vi "Update Registry BK shall be removed later.vi"() -> ()   [LabVIEW 2014]
uses:
  TypeDef/state.ctl
  TypeDef/Qmessage.ctl
  <vilib>/Utility/config.llb/Read Key (Path).vi
  <vilib>/Utility/file.llb/Read From Spreadsheet File (string).vi
  <vilib>/Utility/config.llb/Write Key (Path).vi
  <vilib>/Utility/config.llb/Read Key (String).vi
  <vilib>/Utility/config.llb/NI_LVConfig.lvlib
panel:
  out "ini file path":path
  in  "variation sheet":path caption="Variation Sheet (*.ini)"
  in  "Push":bool
  in  "Help Button":bool
  in  "Run":bool
  in  "Initialize":bool
  out "Status bar":string
  in  "Register change":bool
  in  "Add comment":bool
  in  "View":bool
  in  "NV 31":string
  in  "NV 30":string
  in  "NV 29":string
  in  "NV 28":string
  in  "NV 27":string
  in  "NV 26":string
  in  "NV 25":string
  in  "NV 24":string
  in  "NV 23":string
  in  "NV 22":string
  in  "NV 21":string
  in  "NV 20":string
  in  "NV 19":string
  in  "NV 18":string
  in  "NV 17":string
  in  "NV 16":string
  in  "NV 15":string
  in  "NV 14":string
  in  "NV 13":string
  in  "NV 12":string
  in  "NV 11":string
  in  "NV 10":string
  in  "NV 9":string
  in  "NV 8":string
  in  "NV 7":string
  in  "NV 6":string
  in  "NV 5":string
  in  "NV 4":string
  in  "NV 3":string
  in  "NV 2":string
  in  "NV 1":string
  out "V 31":string
  out "V 30":string
  out "V 29":string
  out "V 28":string
  out "V 27":string
  out "V 26":string
  out "V 25":string
  out "V 24":string
  out "V 23":string
  out "V 22":string
  out "V 21":string
  out "V 20":string
  out "V 19":string
  out "V 18":string
  out "V 17":string
  out "V 16":string
  out "V 15":string
  out "V 14":string
  out "V 13":string
  out "V 12":string
  out "V 11":string
  out "V 10":string
  out "V 9":string
  out "V 8":string
  out "V 7":string
  out "V 6":string
  out "V 5":string
  out "V 4":string
  out "V 3":string
  out "V 2":string
  out "V 1":string
  in  "tdms path":path caption="Variation Registry (*.tdms)"
  in  "Config Path":path caption="Config Path (*.txt)"
  out "N 31":string
  out "N 30":string
  out "N 29":string
  out "N 28":string
  out "N 27":string
  out "N 26":string
  out "N 25":string
  out "N 24":string
  out "N 23":string
  out "N 22":string
  out "N 21":string
  out "N 20":string
  out "N 19":string
  out "N 18":string
  out "N 17":string
  out "N 16":string
  out "N 15":string
  out "N 14":string
  out "N 13":string
  out "N 12":string
  out "N 11":string
  out "N 10":string
  out "N 9":string
  out "N 8":string
  out "N 7":string
  out "N 6":string
  out "N 5":string
  out "N 4":string
  out "N 3":string
  out "N 2":string
  out "N 1":string
  in  "Exit":bool
  # "Update Registry"
  # "Current Configuration"
  # "New Configuration"
  # "Component Name"
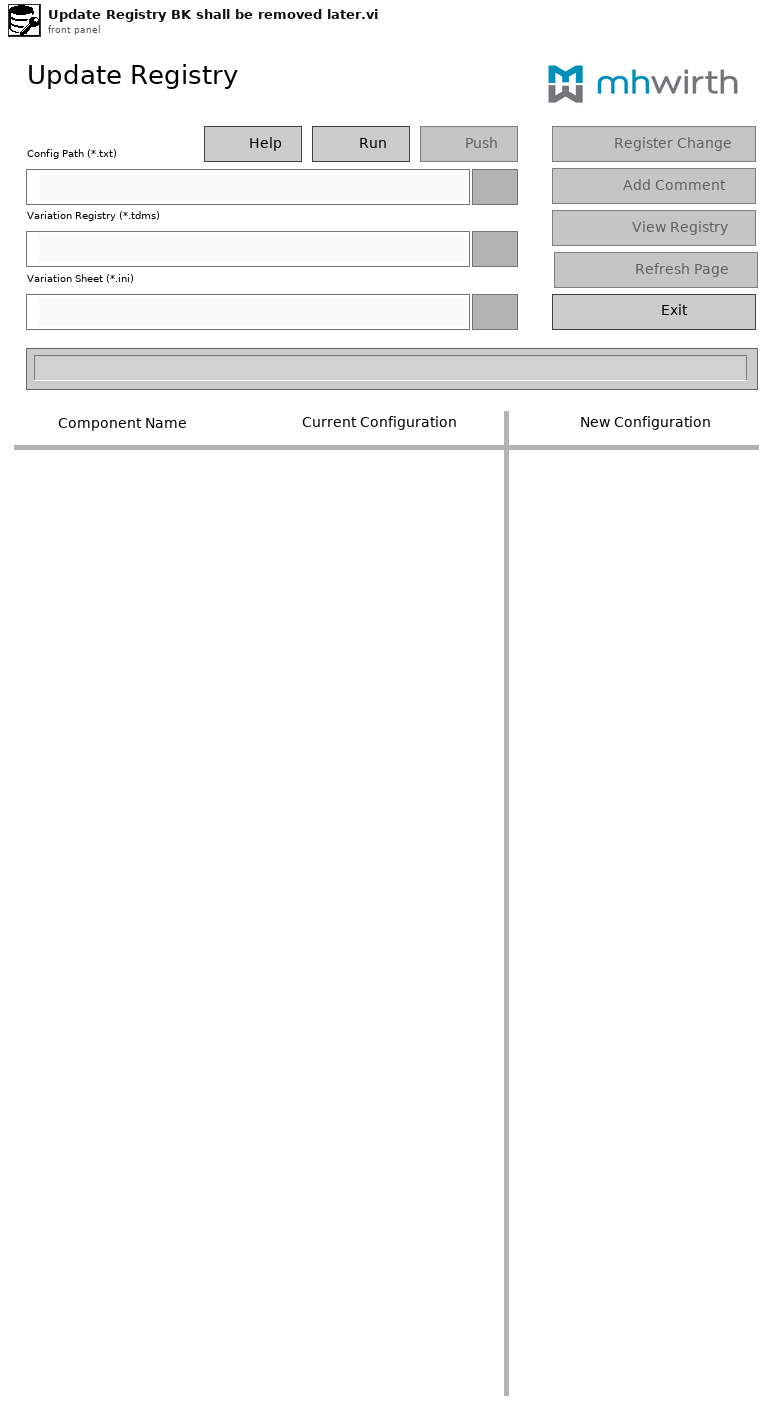
[diagram p1: front panel]
types:
  T1 = cluster{"Folder Path containing version information":path, "File name (including .ini)":path, "Section":string}
  T2 = typedef "Qmessage.ctl" = cluster{"data":variant, "state":T3}
  T3 = typedef "state.ctl" = enum16{"Run", "Initialize 1", "Initialize 2", "Read config file", "Read TDMS", "Config file Error", "Idle", "Update Comp Names", "Update Current Versions", "Make new configuration", "Register Change", "View Registry", "Add Comment", "No New Update", "Check current versions", "Read ini file", "Write ini file", "Read Variation Sheet", "Search and write current versions", "Close"}
  T4 = enum32{"invalid app kind", "Development System", "Run Time System", "Student Edition", "Embedded LabVIEW", "Evaluation", "Custom"}
  T5 = cluster{"keys":refnum<vi>[], "Names":refnum<vi>[], "Current Versions":refnum<vi>[], "New Versions":refnum<vi>[]}
  T6 = cluster{"path":path, "This VI":refnum<vi>, "Level of Application":u8}
  T7 = enum8{"Enabled", "Disabled", "Disabled and Grayed Out"}
  T8 = typedef "NI_LVConfig.lvlib/Config Data RefNum.ctl" = refnum<k1>
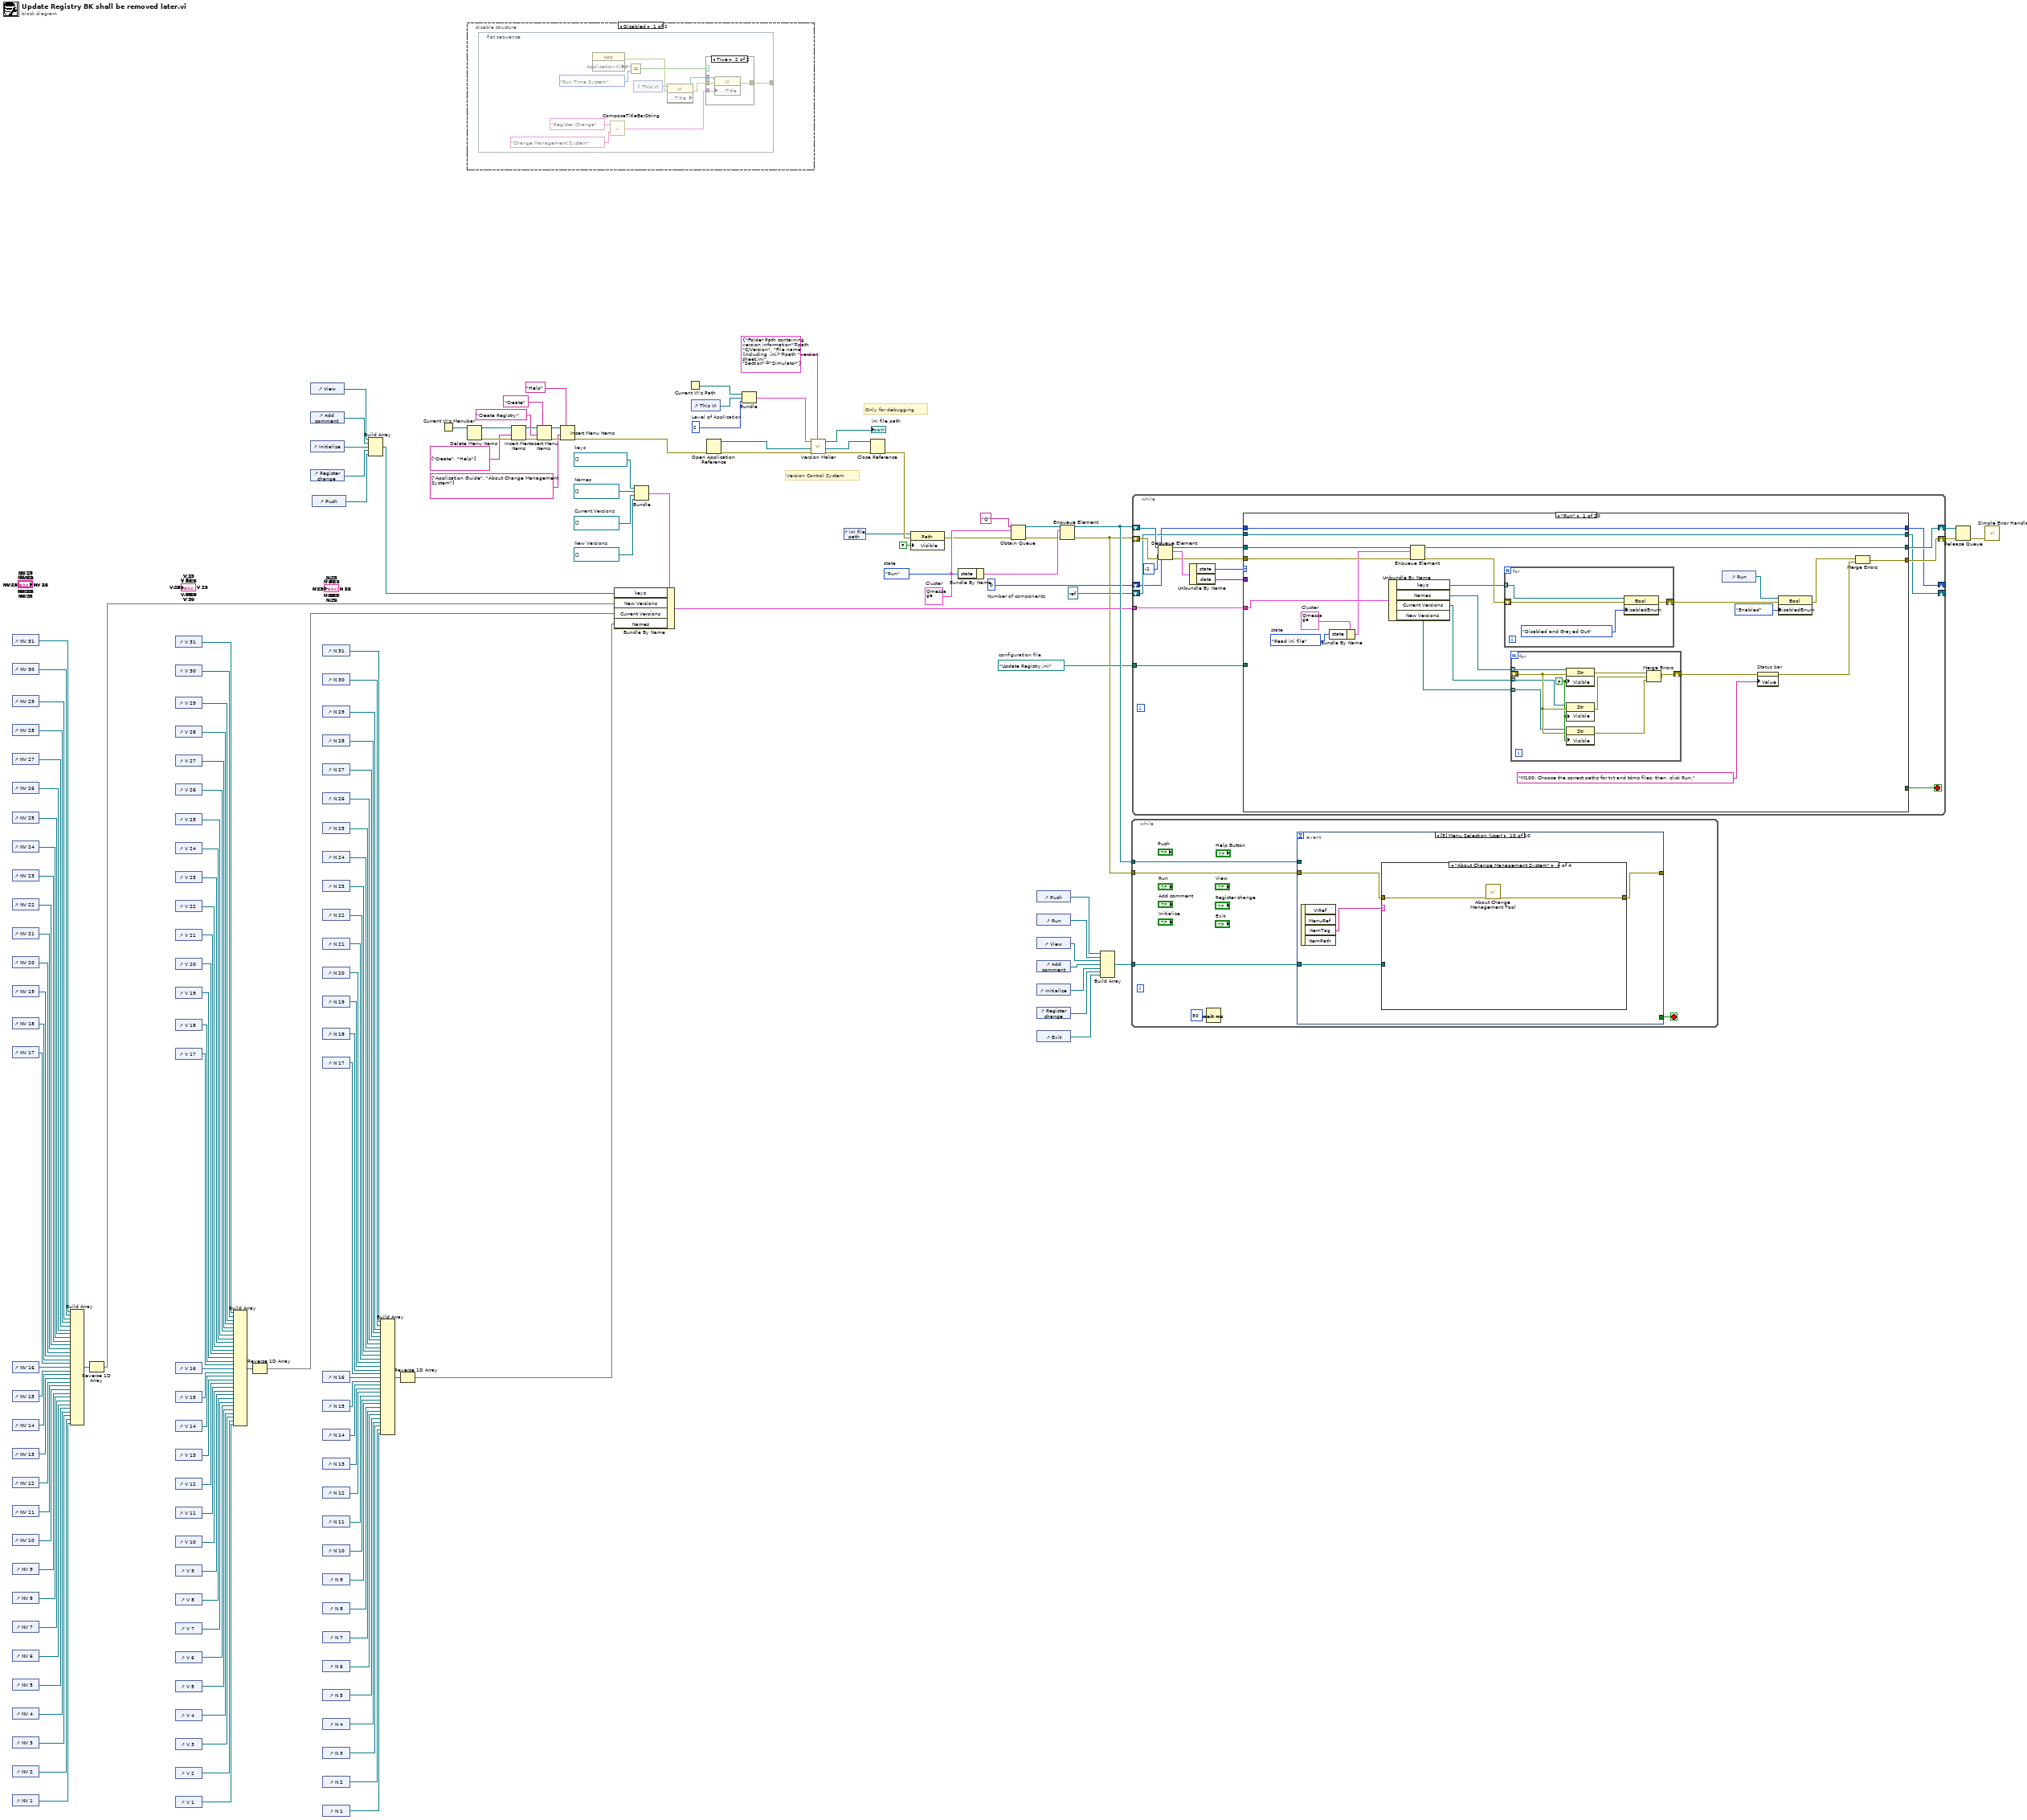
[diagram p0: block diagram]
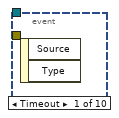
[diagram p4: hidden frame]
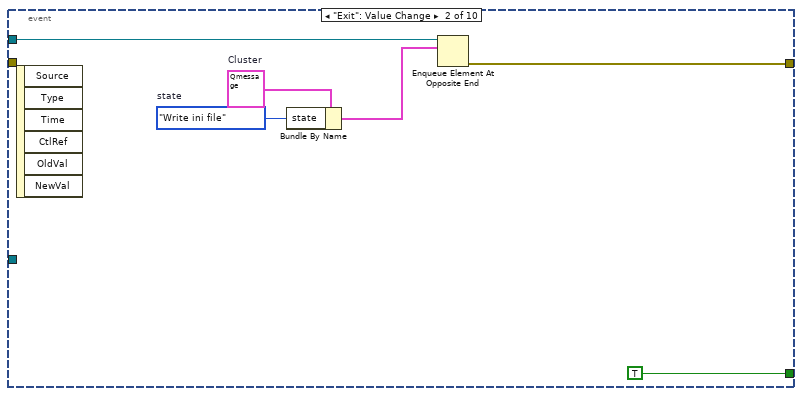
[diagram p5: hidden frame]
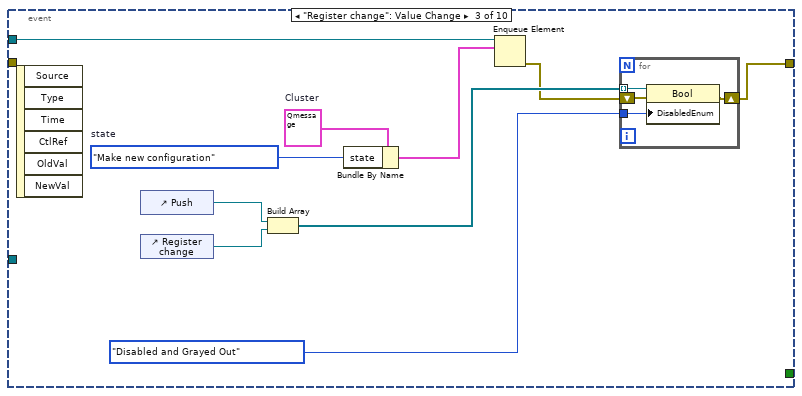
[diagram p6: hidden frame]
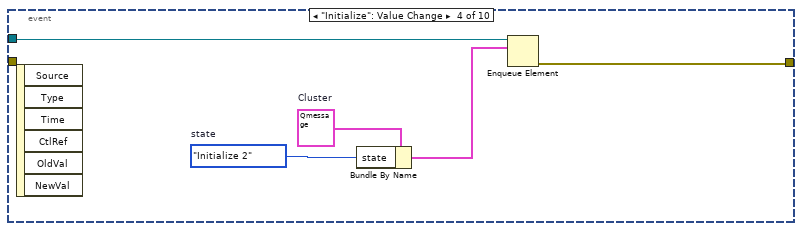
[diagram p7: hidden frame]
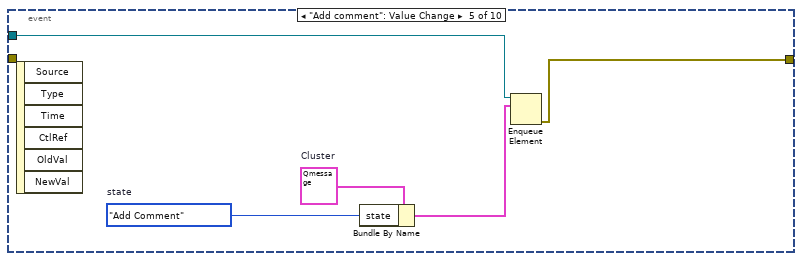
[diagram p8: hidden frame]
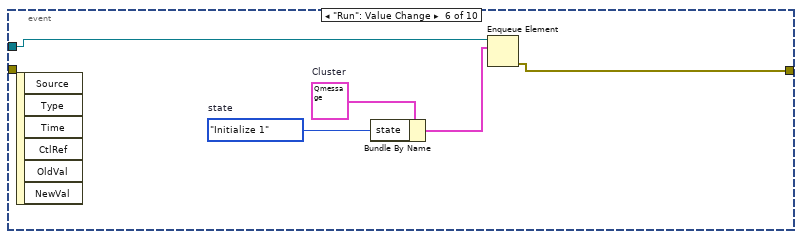
[diagram p9: hidden frame]
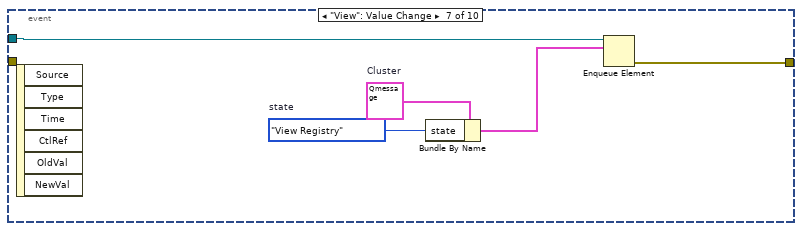
[diagram p10: hidden frame]
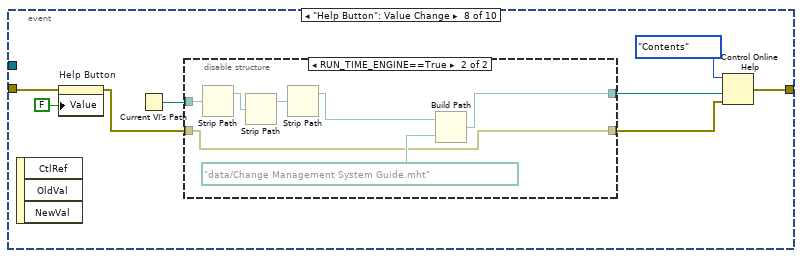
[diagram p11: hidden frame]
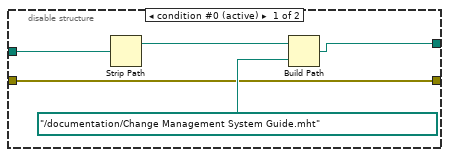
[diagram p12: hidden frame]
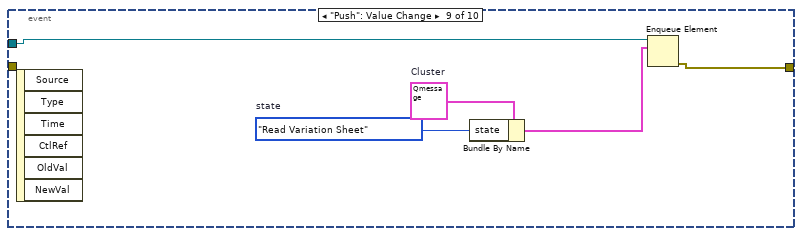
[diagram p13: hidden frame]
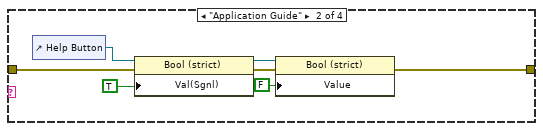
[diagram p15: hidden frame]
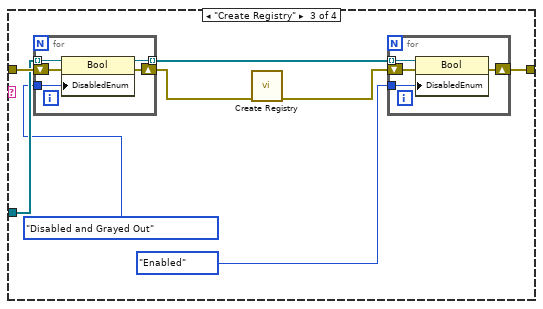
[diagram p16: hidden frame]
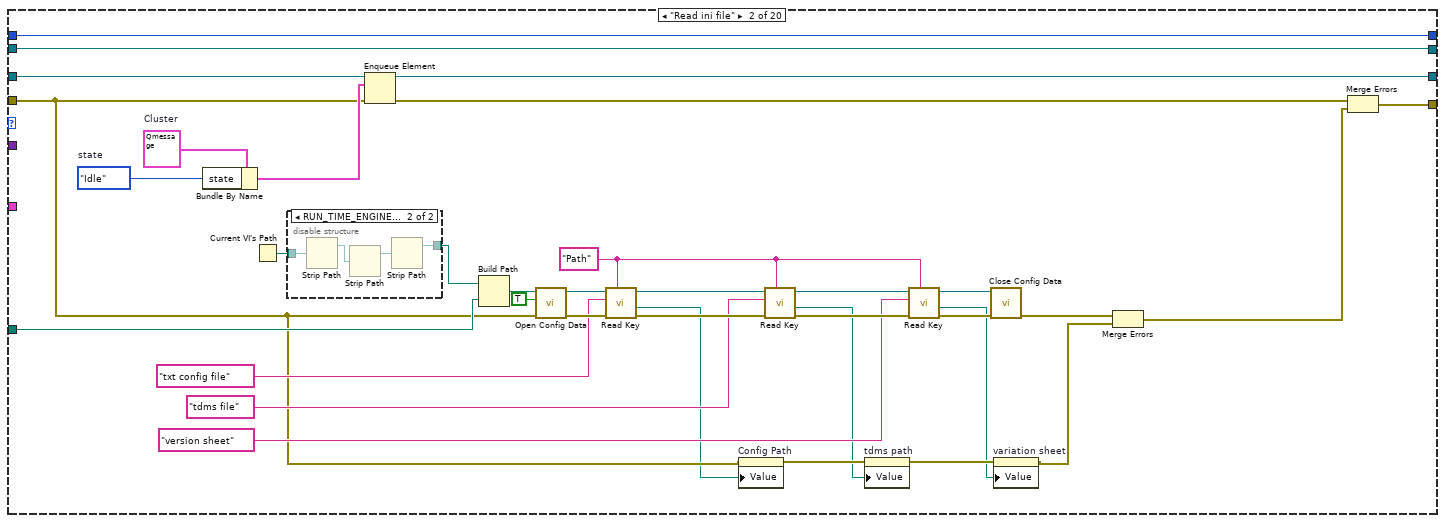
[diagram p17: hidden frame]
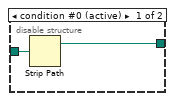
[diagram p18: hidden frame]
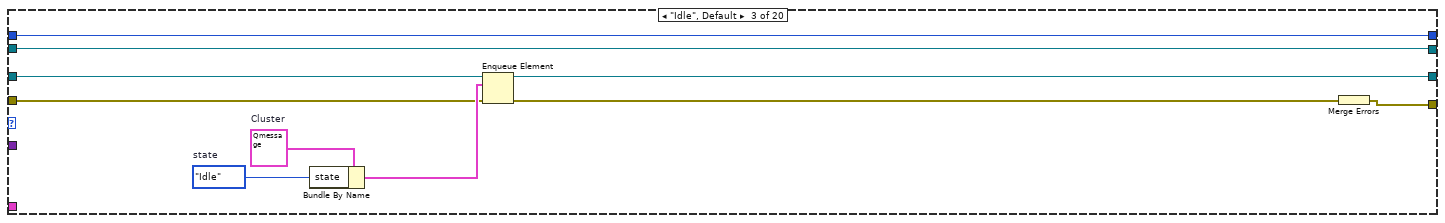
[diagram p19: hidden frame]
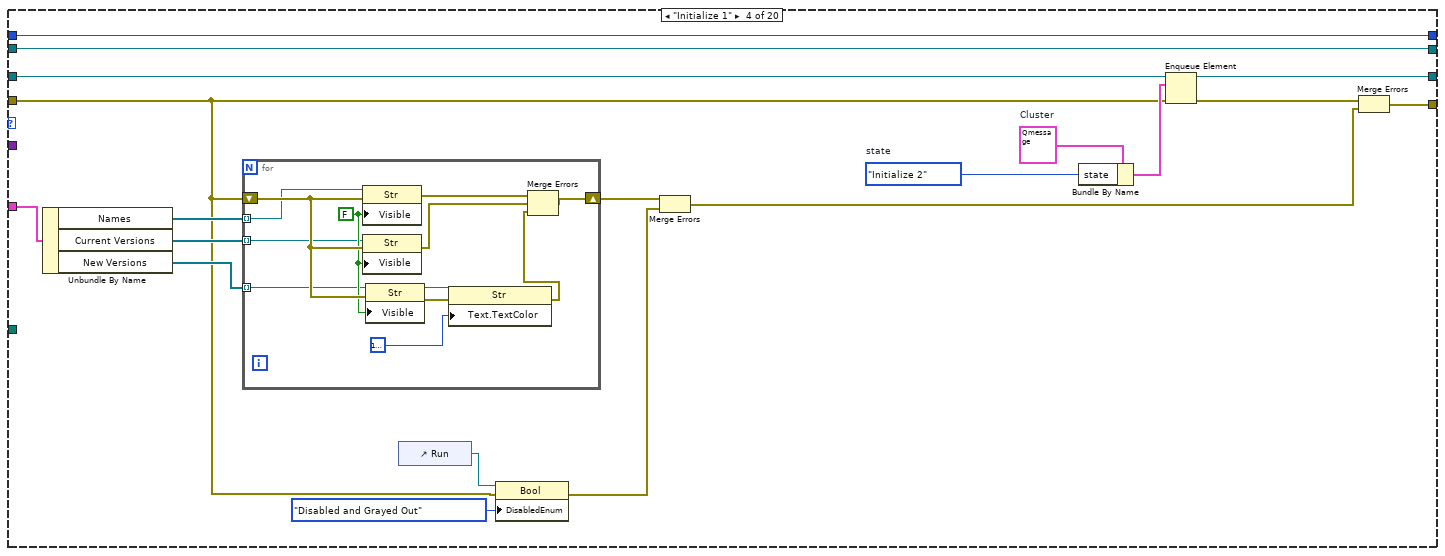
[diagram p20: hidden frame]
diagram:
  w25 = u8 2  # Level of Application
  w37 = path "Update Registry.ini"  # configuration file
  w52 = refnum<vi>[] []  # keys
  w57 = 0  # Number of components
  w49 = refnum<vi>[] []  # New Versions
  w50 = refnum<vi>[] []  # Current Versions
  w51 = refnum<vi>[] []  # Names
  w157 = T2 {"data"=variant, "state"=enum."Initialize 1"}  # Cluster
  w160 = state."Run"  # state
  # "Only for debugging"
  # "Version Control System"
  n1 = control-ref of="NV 31"() -> (w90:refnum<vi>)
  n2 = control-ref of="NV 30"() -> (w89:refnum<vi>)
  n3 = control-ref of="NV 29"() -> (w88:refnum<vi>)
  n4 = control-ref of="NV 28"() -> (w87:refnum<vi>)
  n5 = control-ref of="NV 27"() -> (w86:refnum<vi>)
  n6 = control-ref of="NV 26"() -> (w85:refnum<vi>)
  n7 = control-ref of="NV 25"() -> (w84:refnum<vi>)
  n8 = control-ref of="NV 24"() -> (w83:refnum<vi>)
  n9 = control-ref of="NV 23"() -> (w82:refnum<vi>)
  n10 = control-ref of="NV 22"() -> (w81:refnum<vi>)
  n11 = control-ref of="NV 21"() -> (w80:refnum<vi>)
  n12 = control-ref of="NV 20"() -> (w79:refnum<vi>)
  n13 = control-ref of="NV 19"() -> (w78:refnum<vi>)
  n14 = control-ref of="NV 18"() -> (w77:refnum<vi>)
  n15 = control-ref of="NV 17"() -> (w76:refnum<vi>)
  n16 = control-ref of="NV 16"() -> (w75:refnum<vi>)
  n17 = control-ref of="NV 15"() -> (w74:refnum<vi>)
  n18 = control-ref of="NV 14"() -> (w73:refnum<vi>)
  n19 = control-ref of="NV 13"() -> (w72:refnum<vi>)
  n20 = control-ref of="NV 12"() -> (w71:refnum<vi>)
  n21 = control-ref of="NV 11"() -> (w70:refnum<vi>)
  n22 = control-ref of="NV 10"() -> (w69:refnum<vi>)
  n23 = control-ref of="NV 9"() -> (w68:refnum<vi>)
  n24 = control-ref of="NV 8"() -> (w67:refnum<vi>)
  n25 = control-ref of="NV 7"() -> (w66:refnum<vi>)
  n26 = control-ref of="NV 6"() -> (w65:refnum<vi>)
  n27 = control-ref of="NV 5"() -> (w64:refnum<vi>)
  n28 = control-ref of="NV 4"() -> (w63:refnum<vi>)
  n29 = control-ref of="NV 3"() -> (w62:refnum<vi>)
  n30 = control-ref of="NV 2"() -> (w61:refnum<vi>)
  n31 = control-ref of="NV 1"() -> (w60:refnum<vi>)
  n32 = Build Array(w90, w89, w88, w87, w86, w85, w84, w83, w82, w81, w80, w79, w78, w77, w76, w75, w74, w73, w72, w71, w70, w69, w68, w67, w66, w65, w64, w63, w62, w61, w60) -> (w59:refnum<vi>[])
  n33 = Reverse 1D Array(array=w59) -> (reversed array=w43:refnum<vi>[])
  n34 = control-ref of="V 31"() -> (w122:refnum<vi>)
  n35 = control-ref of="V 30"() -> (w121:refnum<vi>)
  n36 = control-ref of="V 29"() -> (w120:refnum<vi>)
  n37 = control-ref of="V 28"() -> (w119:refnum<vi>)
  n38 = control-ref of="V 27"() -> (w118:refnum<vi>)
  n39 = control-ref of="V 26"() -> (w117:refnum<vi>)
  n40 = control-ref of="V 25"() -> (w116:refnum<vi>)
  n41 = control-ref of="V 24"() -> (w115:refnum<vi>)
  n42 = control-ref of="V 23"() -> (w114:refnum<vi>)
  n43 = control-ref of="V 22"() -> (w113:refnum<vi>)
  n44 = control-ref of="V 21"() -> (w112:refnum<vi>)
  n45 = control-ref of="V 20"() -> (w111:refnum<vi>)
  n46 = control-ref of="V 19"() -> (w110:refnum<vi>)
  n47 = control-ref of="V 18"() -> (w109:refnum<vi>)
  n48 = control-ref of="V 17"() -> (w108:refnum<vi>)
  n49 = control-ref of="V 16"() -> (w107:refnum<vi>)
  n50 = control-ref of="V 15"() -> (w106:refnum<vi>)
  n51 = control-ref of="V 14"() -> (w105:refnum<vi>)
  n52 = control-ref of="V 13"() -> (w104:refnum<vi>)
  n53 = control-ref of="V 12"() -> (w103:refnum<vi>)
  n54 = control-ref of="V 11"() -> (w102:refnum<vi>)
  n55 = control-ref of="V 10"() -> (w101:refnum<vi>)
  n56 = control-ref of="V 9"() -> (w100:refnum<vi>)
  n57 = control-ref of="V 8"() -> (w99:refnum<vi>)
  n58 = control-ref of="V 7"() -> (w98:refnum<vi>)
  n59 = control-ref of="V 6"() -> (w97:refnum<vi>)
  n60 = control-ref of="V 5"() -> (w96:refnum<vi>)
  n61 = control-ref of="V 4"() -> (w95:refnum<vi>)
  n62 = control-ref of="V 3"() -> (w94:refnum<vi>)
  n63 = control-ref of="V 2"() -> (w93:refnum<vi>)
  n64 = control-ref of="V 1"() -> (w92:refnum<vi>)
  n65 = Build Array(w122, w121, w120, w119, w118, w117, w116, w115, w114, w113, w112, w111, w110, w109, w108, w107, w106, w105, w104, w103, w102, w101, w100, w99, w98, w97, w96, w95, w94, w93, w92) -> (w91:refnum<vi>[])
  n66 = Reverse 1D Array(array=w91) -> (reversed array=w44:refnum<vi>[])
  n67 = control-ref of="View"() -> (w56:refnum<vi>)
  n68 = control-ref of="Add comment"() -> (w55:refnum<vi>)
  n69 = control-ref of="Initialize"() -> (w54:refnum<vi>)
  n70 = control-ref of="Register change"() -> (w53:refnum<vi>)
  n71 = control-ref of="Push"() -> (w38:refnum<vi>)
  n72 = control-ref of="N 31"() -> (w155:refnum<vi>)
  n73 = control-ref of="N 30"() -> (w154:refnum<vi>)
  n74 = control-ref of="N 29"() -> (w153:refnum<vi>)
  n75 = control-ref of="N 28"() -> (w152:refnum<vi>)
  n76 = control-ref of="N 27"() -> (w151:refnum<vi>)
  n77 = control-ref of="N 26"() -> (w150:refnum<vi>)
  n78 = control-ref of="N 25"() -> (w149:refnum<vi>)
  n79 = control-ref of="N 24"() -> (w148:refnum<vi>)
  n80 = control-ref of="N 23"() -> (w147:refnum<vi>)
  n81 = control-ref of="N 22"() -> (w146:refnum<vi>)
  n82 = control-ref of="N 21"() -> (w145:refnum<vi>)
  n83 = control-ref of="N 20"() -> (w144:refnum<vi>)
  n84 = control-ref of="N 19"() -> (w143:refnum<vi>)
  n85 = control-ref of="N 18"() -> (w142:refnum<vi>)
  n86 = control-ref of="N 17"() -> (w141:refnum<vi>)
  n87 = control-ref of="N 16"() -> (w140:refnum<vi>)
  n88 = control-ref of="N 15"() -> (w139:refnum<vi>)
  n89 = control-ref of="N 14"() -> (w138:refnum<vi>)
  n90 = control-ref of="N 13"() -> (w137:refnum<vi>)
  n91 = control-ref of="N 12"() -> (w136:refnum<vi>)
  n92 = control-ref of="N 11"() -> (w135:refnum<vi>)
  n93 = control-ref of="N 10"() -> (w134:refnum<vi>)
  n94 = control-ref of="N 9"() -> (w133:refnum<vi>)
  n95 = control-ref of="N 8"() -> (w132:refnum<vi>)
  n96 = control-ref of="N 7"() -> (w131:refnum<vi>)
  n97 = control-ref of="N 6"() -> (w130:refnum<vi>)
  n98 = control-ref of="N 5"() -> (w129:refnum<vi>)
  n99 = control-ref of="N 4"() -> (w128:refnum<vi>)
  n100 = control-ref of="N 3"() -> (w127:refnum<vi>)
  n101 = control-ref of="N 2"() -> (w126:refnum<vi>)
  n102 = control-ref of="N 1"() -> (w125:refnum<vi>)
  n103 = Build Array(w56, w55, w54, w53, w38) -> (w46:refnum<vi>[])
  n104 = Build Array(w155, w154, w153, w152, w151, w150, w149, w148, w147, w146, w145, w144, w143, w142, w141, w140, w139, w138, w137, w136, w135, w134, w133, w132, w131, w130, w129, w128, w127, w126, w125) -> (w124:refnum<vi>[])
  n105 = Reverse 1D Array(array=w124) -> (reversed array=w45:refnum<vi>[])
  n106 = Current VI's Menubar() -> (w22:refnum<k9>)
  n107 = disable-structure shown="Disabled" {
    frame Disabled {
      n108 = flat-sequence {
        tunnel: [w161] -> _
        frame #0 {
          n109 = property on="Property Node" class="App"() -> (error out=w163:errorcluster, "Application:Kind"=w169:T4)  [unwired: 2 in, 1 out]
          n110 = call "ComposeTitleBarString.vi"("ProjectName"="Change Management System" ("Application"), "Application"="Register Change") -> ("TitleBar"=w171:string)
          n111 = Equal?(x=w169, y=T4."Run Time System" ("Applikation:Typ")) -> (x = y?=w170:bool)
          n112 = control-ref of="This VI"() -> (w167:refnum<vi>)
          n113 = property on="Property Node" class="VI" props=["Front Panel.Title"](reference=w167, error in=w163) -> (reference out=w166:refnum<vi>, error out=w162:errorcluster)  [unwired: 1 out]
          n114 = case shown="True" w170 {
            tunnel: w171 -> [_ w176]
            tunnel: w166 -> [_ w175]
            tunnel: w162 -> [w172 w174]
            tunnel: [w172 w173] -> w161
            frame False {
            }
            frame True {
              n115 = property class="VI"(reference=w175, error in=w174, "Front Panel.Title"=w176) -> (error out=w173:errorcluster)  [unwired: 1 out]
            }
          }
        }
      }
    }
    frame Enabled {
    }
  }
  n116 = Delete Menu Items(9:w22) -> (0:w21:errorcluster, 3:w20:refnum<k9>)  [unwired: 3 in]
  n117 = Insert Menu Items(6:w21, 7:string[] ["Create", "Help"] ("item tags"), 9:w20) -> (0:w16:errorcluster, 3:w18:refnum<k9>)  [unwired: 3 in, 1 out]
  n118 = Insert Menu Items(5:"Create", 6:w16, 7:"Create Registry", 9:w18) -> (0:w15:errorcluster, 3:w14:refnum<k9>)  [unwired: 2 in, 1 out]
  n119 = Insert Menu Items(5:"Help", 6:w15, 7:string[] ["Application Guide", "About Change Management System"] ("item tags"), 9:w14) -> (0:w10:errorcluster)  [unwired: 2 in, 2 out]
  n120 = Bundle("keys"=w52, "Names"=w51, "Current Versions"=w50, "New Versions"=w49) -> (w47:T5)  [unwired: 1 in]
  n121 = Bundle By Name(cluster=w47, "keys"=w46, "New Versions"=w43, "Current Versions"=w44, "Names"=w45) -> (w48:T5)
  n122 = Current VI's Path() -> (path=w23:path)
  n123 = control-ref of="This VI"() -> (w24:refnum<vi>)
  n124 = Open Application Reference(8:w10) -> (0:w36:errorcluster, 3:w32:refnum<vi>)  [unwired: 3 in]
  n125 = Bundle("path"=w23, "This VI"=w24, "Level of Application"=w25) -> (w26:T6)  [unwired: 1 in]
  n126 = call "Version Maker.vi"("Version Sheet Cluster"=T1 {"Folder Path containing version information"=path "C:/Version", "File name (including .ini)"=path "version sheet.ini", "Section"="Simulator"}, "Error In"=w36, "Open Application Reference in"=w32, "VI Information"=w26) -> ("Error Out"=w35:errorcluster, "Open Application Reference out"=w31:refnum<vi>, "ini file path"=→"ini file path":path)  [unwired: 5 in]
  n127 = control-ref of="ini file path"() -> (w28:refnum<vi>)
  n128 = Close Reference(reference=w31, error in (no error)=w35) -> (error out=w29:errorcluster)
  n129 = property class="Path"(reference=w28, error in=w29, "Visible"=FALSE) -> (error out=w30:errorcluster)  [unwired: 1 out]
  n130 = Bundle By Name(cluster=w157, "state"=w160) -> (w156:T2)
  n131 = Obtain Queue(name (unnamed)="Q", element data type=w157, error in (no error)=w30) -> (queue out=w159:refnum<queue>, error out=w42:errorcluster)  [unwired: 2 in, 1 out]
  n132 = control-ref of="Push"() -> (w8:refnum<vi>)
  n133 = control-ref of="Run"() -> (w7:refnum<vi>)
  n134 = control-ref of="View"() -> (w6:refnum<vi>)
  n135 = control-ref of="Add comment"() -> (w5:refnum<vi>)
  n136 = control-ref of="Initialize"() -> (w4:refnum<vi>)
  n137 = control-ref of="Register change"() -> (w3:refnum<vi>)
  n138 = control-ref of="Exit"() -> (w2:refnum<vi>)
  n139 = Enqueue Element(queue=w159, element=w156, error in (no error)=w42) -> (queue out=w123:refnum<queue>, error out=w9:errorcluster)  [unwired: 1 in, 1 out]
  n140 = Build Array(w8, w7, w6, w5, w4, w3, w2) -> (w1:refnum<vi>[])
  n141 = while {
    tunnel: w123 -> [w180]
    tunnel: w9 -> [w178]
    tunnel: w1 -> [w177]
    stop <- w179 stop-if-true
    n142 = Wait (ms)(milliseconds to wait=u32 50) -> ()  [unwired: 1 out]
    n143 = event shown="[9] Menu Selection (User)" {
      selector: _ -> [_ _ _ _ _ _ _ _ _ _]
      dyn-events: _ -> [_ _ _ _ _ _ _ _ _ _]
      timeout: _ -> [_ _ _ _ _ _ _ _ _ _]
      tunnel: w180 -> [_ w184 w195 w203 w211 w214 w218 _ w243 _]
      tunnel: [_ TRUE _ _ _ _ _ _ _ _] -> w179
      tunnel: [_ w182 w188 w202 w207 w212 w217 w228 w242 w248] -> _
      tunnel: w178 -> [_ _ _ _ _ _ _ w224 _ w249]
      tunnel: w177 -> [_ _ _ _ _ _ _ _ _ w247]
      event Timeout {
        n144 = event-data() -> ()  [unwired: 1 in, 2 out]
      }
      event "Exit": Value Change {
        w187 = T2 {"data"=variant, "state"=enum."Initialize 1"}  # Cluster
        w186 = state."Write ini file"  # state
        n145 = event-data() -> ()  [unwired: 1 in, 6 out]
        n146 = Bundle By Name(cluster=w187, "state"=w186) -> (w185:T2)
        n147 = Enqueue Element At Opposite End(queue=w184, element=w185) -> (error out=w182:errorcluster)  [unwired: 2 in, 2 out]
      }
      event "Register change": Value Change {
        w197 = T2 {"data"=variant, "state"=enum."Initialize 1"}  # Cluster
        w194 = state."Make new configuration"  # state
        n148 = event-data() -> ()  [unwired: 1 in, 6 out]
        n149 = control-ref of="Push"() -> (w193:refnum<vi>)
        n150 = control-ref of="Register change"() -> (w192:refnum<vi>)
        n151 = Build Array(w193, w192) -> (w191:refnum<vi>[])
        n152 = Bundle By Name(cluster=w197, "state"=w194) -> (w196:T2)
        n153 = Enqueue Element(queue=w195, element=w196) -> (error out=w189:errorcluster)  [unwired: 2 in, 2 out]
        n154 = for {
          tunnel: w191 -> [w201] mode=indexing
          tunnel: T7."Disabled and Grayed Out" ("Disabled") -> [w200]
          shift-right: [w198] -> w188
          shift-left: w189 -> [w199]
          n155 = property class="Bool"(reference=w201, error in=w199, "DisabledEnum"=w200) -> (error out=w198:errorcluster)  [unwired: 1 out]
        }
      }
      event "Initialize": Value Change {
        w206 = T2 {"data"=variant, "state"=enum."Initialize 1"}  # Cluster
        w204 = state."Initialize 2"  # state
        n156 = event-data() -> ()  [unwired: 1 in, 6 out]
        n157 = Bundle By Name(cluster=w206, "state"=w204) -> (w205:T2)
        n158 = Enqueue Element(queue=w203, element=w205) -> (error out=w202:errorcluster)  [unwired: 2 in, 2 out]
      }
      event "Add comment": Value Change {
        w209 = T2 {"data"=variant, "state"=enum."Initialize 1"}  # Cluster
        w208 = state."Add Comment"  # state
        n159 = event-data() -> ()  [unwired: 1 in, 6 out]
        n160 = Bundle By Name(cluster=w209, "state"=w208) -> (w210:T2)
        n161 = Enqueue Element(queue=w211, element=w210) -> (error out=w207:errorcluster)  [unwired: 2 in, 2 out]
      }
      event "Run": Value Change {
        w216 = T2 {"data"=variant, "state"=enum."Initialize 1"}  # Cluster
        w215 = state."Initialize 1"  # state
        n162 = event-data() -> ()  [unwired: 1 in, 6 out]
        n163 = Bundle By Name(cluster=w216, "state"=w215) -> (w213:T2)
        n164 = Enqueue Element(queue=w214, element=w213) -> (error out=w212:errorcluster)  [unwired: 2 in, 2 out]
      }
      event "View": Value Change {
        w221 = T2 {"data"=variant, "state"=enum."Initialize 1"}  # Cluster
        w220 = state."View Registry"  # state
        n165 = event-data() -> ()  [unwired: 1 in, 6 out]
        n166 = Bundle By Name(cluster=w221, "state"=w220) -> (w219:T2)
        n167 = Enqueue Element(queue=w218, element=w219) -> (error out=w217:errorcluster)  [unwired: 2 in, 2 out]
      }
      event "Help Button": Value Change {
        n168 = event-data() -> ()  [unwired: 1 in, 3 out]
        n169 = property on="Help Button" class="Bool (strict)"(error in=w224, "Value"=FALSE ("Help Button")) -> (error out=w223:errorcluster)  [unwired: 1 in, 1 out]
        n170 = Current VI's Path() -> (path=w227:path)
        n171 = disable-structure shown="RUN_TIME_ENGINE==True" {
          disable-tunnel: w227 -> [w234 w241]
          disable-tunnel: [w231 w237] -> w226
          disable-tunnel: w223 -> [w230 w235]
          disable-tunnel: [w230 w235] -> w222
          frame condition #0 (active) {
            n172 = Strip Path(path=w234) -> (stripped path=w233:path)  [unwired: 1 out]
            n173 = Build Path(base path=w233, name or relative path=path "../documentation/Change Management System Guide.mht") -> (appended path=w231:path)
          }
          frame condition #1 {
            n174 = Strip Path(path=w241) -> (stripped path=w240:path)  [unwired: 1 out]
            n175 = Strip Path(path=w240) -> (stripped path=w239:path)  [unwired: 1 out]
            n176 = Strip Path(path=w239) -> (stripped path=w236:path)  [unwired: 1 out]
            n177 = Build Path(base path=w236, name or relative path=path "data/Change Management System Guide.mht") -> (appended path=w237:path)
          }
        }
        n178 = Control Online Help(1:w222, 2:w226, 4:enum16{"Contents", "Key", "Close"}."Contents" ("Operation")) -> (0:w228:errorcluster)  [unwired: 1 in]
      }
      event "Push": Value Change {
        w246 = T2 {"data"=variant, "state"=enum."Initialize 1"}  # Cluster
        w245 = state."Read Variation Sheet"  # state
        n179 = event-data() -> ()  [unwired: 1 in, 6 out]
        n180 = Bundle By Name(cluster=w246, "state"=w245) -> (w244:T2)
        n181 = Enqueue Element(queue=w243, element=w244) -> (error out=w242:errorcluster)  [unwired: 2 in, 2 out]
      }
      event Menu Selection (User) {
        n182 = event-data() -> ("ItemTag"=w250:string)  [unwired: 1 in, 3 out]
        n183 = case shown="\"About Change Management System\"" w250 {
          tunnel: w249 -> [w251 w253 w266 w277]
          tunnel: [w251 w252 w259 w276] -> w248
          tunnel: w247 -> [_ _ w265 _]
          frame "default", Default {
          }
          frame "Application Guide" {
            n184 = control-ref of="Help Button"() -> (w258:refnum<vi>)
            n185 = property class="Bool (strict)"(reference=w258, error in=w253, "Val(Sgnl)"=TRUE) -> (reference out=w256:refnum<vi>, error out=w255:errorcluster)
            n186 = property class="Bool (strict)"(reference=w256, error in=w255, "Value"=FALSE ("Value (Signaling)")) -> (error out=w252:errorcluster)  [unwired: 1 out]
          }
          frame "Create Registry" {
            n187 = for {
              tunnel: w265 -> [w274] mode=indexing
              tunnel: T7."Disabled and Grayed Out" ("Disabled") -> [w273]
              tunnel: [w272] -> w263 mode=indexing
              shift-right: [w271] -> w261
              shift-left: w266 -> [w275]
              n188 = property class="Bool"(reference=w274, error in=w275, "DisabledEnum"=w273) -> (reference out=w272:refnum<vi>, error out=w271:errorcluster)
            }
            n189 = call "Create Registry.vi"("Error In"=w261) -> ("Error Out"=w260:errorcluster)  [unwired: 10 in]
            n190 = for {
              tunnel: w263 -> [w269] mode=indexing
              tunnel: T7."Enabled" ("Disabled") -> [w268]
              shift-right: [w267] -> w259
              shift-left: w260 -> [w270]
              n191 = property class="Bool"(reference=w269, error in=w270, "DisabledEnum"=w268) -> (error out=w267:errorcluster)  [unwired: 1 out]
            }
          }
          frame "About Change Management System" {
            n192 = call "About Change Management Tool.vi"("Error In"=w277) -> ("Error Out"=w276:errorcluster)  [unwired: 10 in]
          }
        }
      }
    }
  }
  n193 = while {
    shift-right: [w288] -> w40
    shift-left: w123 -> [w292]
    shift-right: [w287] -> w41
    shift-left: w9 -> [w294]
    tunnel: w48 -> [w283]
    shift-right: [w282] -> _
    shift-left: refnum<k34> refnum ("tdms file out") -> [w281]
    shift-right: [w280] -> _
    shift-left: w57 -> [w279]
    tunnel: w37 -> [w278]
    stop <- w284 stop-if-true
    n194 = Dequeue Element(queue=w292, timeout in ms (-1)=-1, error in (no error)=w294) -> (queue out=w289:refnum<queue>, element=w293:T2, error out=w285:errorcluster)  [unwired: 1 out]
    n195 = Unbundle By Name(w293) -> ("state"=w291:T3, "data"=w290:variant)
    n196 = case shown="\"Run\"" w291 {
      tunnel: w290 -> [_ _ _ _ _ _ _ w526 w549 _ w633 _ _ _ _ _ _ _ _ w862]
      tunnel: w289 -> [w299 w362 w376 w382 w421 w439 w475 w518 w542 w576 w627 w662 w688 w704 w720 w732 w760 w803 w822 w864]
      tunnel: [w298 w361 w375 w381 w420 w438 w475 w518 w542 w576 w627 w662 w688 w704 w720 w732 w759 w803 w821 w864] -> w288
      tunnel: w285 -> [w297 w336 w373 w385 w415 w441 w474 w523 w546 w585 w632 w667 w682 w707 w715 w738 w758 w794 w820 w853]
      tunnel: [w309 w356 w372 w394 w427 w449 w477 w517 w541 w578 w628 w659 w679 w703 w714 w738 w763 w800 w819 w852] -> w287
      tunnel: [_ _ _ _ _ _ _ _ _ _ _ _ _ _ _ _ _ TRUE _ _] -> w284
      tunnel: w283 -> [w314 _ _ w399 w416 _ _ w513 w540 w588 _ _ _ _ w717 _ _ w789 _ w858]
      tunnel: [w316 w364 w380 w389 w422 w445 w473 w511 w537 w589 w629 w668 w685 w709 w719 w734 w777 w797 w835 w863] -> w282
      tunnel: w281 -> [w316 w364 w380 w389 w422 w445 w472 w511 w537 w589 w629 w668 w676 w709 w719 w734 w777 w797 w835 w863]
      tunnel: [w315 w363 w379 w395 w417 w437 w471 w510 w535 w582 w621 w669 w687 w708 w718 w733 w776 w784 w834 w854] -> w280
      tunnel: w279 -> [w315 w363 w379 w395 w417 _ w471 w510 w535 w582 w621 w669 w687 w708 w718 w733 w776 w784 w834 w854]
      tunnel: w278 -> [_ w338 _ _ _ _ _ _ _ _ _ _ _ _ _ _ w743 _ _ _]
      frame "Run" {
        w301 = T2 {"data"=variant, "state"=enum."Initialize 1"}  # Cluster
        w300 = state."Read ini file"  # state
        n197 = Bundle By Name(cluster=w301, "state"=w300) -> (w295:T2)
        n198 = Unbundle By Name(w314) -> ("keys"=w313:refnum<vi>[], "Names"=w312:refnum<vi>[], "Current Versions"=w311:refnum<vi>[], "New Versions"=w310:refnum<vi>[])
        n199 = Enqueue Element(queue=w299, element=w295, error in (no error)=w297) -> (queue out=w298:refnum<queue>, error out=w296:errorcluster)  [unwired: 1 in, 1 out]
        n200 = for {
          shift-right: [w327] -> w306
          shift-left: w296 -> [w328]
          tunnel: w313 -> [w326] mode=indexing
          n201 = property class="Bool"(reference=w326, error in=w328, "DisabledEnum"=T7."Disabled and Grayed Out" ("Disabled")) -> (error out=w327:errorcluster)  [unwired: 1 out]
        }
        n202 = for {
          shift-right: [w325] -> w304
          shift-left: _ -> [w322]
          tunnel: w312 -> [w319] mode=indexing
          tunnel: w311 -> [w318] mode=indexing
          tunnel: w310 -> [w317] mode=indexing
          w321 = FALSE ("Visible")
          n203 = property class="Str"(reference=w319, error in=w322, "Visible"=w321) -> (error out=w324:errorcluster)  [unwired: 1 out]
          n204 = property class="Str"(reference=w318, error in=w322, "Visible"=w321) -> (error out=w323:errorcluster)  [unwired: 1 out]
          n205 = property class="Str"(reference=w317, error in=w322, "Visible"=w321) -> (error out=w320:errorcluster)  [unwired: 1 out]
          n206 = Merge Errors(w324, w323, w320) -> (w325:errorcluster)
        }
        n207 = control-ref of="Run"() -> (w308:refnum<vi>)
        n208 = property on="Status bar" class="Str"(error in=w304, "Value"="M100: Choose the correct paths for txt and tdms files; then, click Run." ("Status bar")) -> (error out=w303:errorcluster)  [unwired: 1 in, 1 out]
        n209 = property class="Bool"(reference=w308, error in=w306, "DisabledEnum"=T7."Enabled" ("Disabled")) -> (error out=w305:errorcluster)  [unwired: 1 out]
        n210 = Merge Errors(w305, w303) -> (w309:errorcluster)
      }
      frame "Read ini file" {
        w339 = "Path" ("section")
        w360 = T2 {"data"=variant, "state"=enum."Initialize 1"}  # Cluster
        w359 = state."Idle"  # state
        n211 = Bundle By Name(cluster=w360, "state"=w359) -> (w358:T2)
        n212 = Current VI's Path() -> (path=w346:path)
        n213 = disable-structure shown="RUN_TIME_ENGINE==True" {
          disable-tunnel: w346 -> [w366 w370]
          disable-tunnel: [w365 w367] -> w345
          frame condition #0 (active) {
            n214 = Strip Path(path=w366) -> (stripped path=w365:path)  [unwired: 1 out]
          }
          frame condition #1 {
            n215 = Strip Path(path=w370) -> (stripped path=w369:path)  [unwired: 1 out]
            n216 = Strip Path(path=w369) -> (stripped path=w368:path)  [unwired: 1 out]
            n217 = Strip Path(path=w368) -> (stripped path=w367:path)  [unwired: 1 out]
          }
        }
        n218 = Enqueue Element(queue=w362, element=w358, error in (no error)=w336) -> (queue out=w361:refnum<queue>, error out=w357:errorcluster)  [unwired: 1 in, 1 out]
        n219 = Build Path(base path=w345, name or relative path=w338) -> (appended path=w355:path)
        n220 = call <vilib>:"Open Config Data.vi"("error in (no error)"=w336, "create file if necessary (T)"=TRUE, "configuration file path"=w355) -> ("error out"=w353:errorcluster, "refnum"=w354:T8)  [unwired: 6 in, 1 out]
        n221 = call-poly <vilib>:"Read Key.vi"("section"=w339, "error in (no error)"=w353, "key"="txt config file", "refnum"=w354) -> ("error out"=w351:errorcluster, "value"=w335:path, "refnum out"=w350:T8)  [unwired: 4 in, 1 out]
        n222 = property on="Config Path" class="Path"(error in=w336, "Value"=w335) -> (error out=w334:errorcluster)  [unwired: 1 in, 1 out]
        n223 = call-poly <vilib>:"Read Key.vi"("section"=w339, "error in (no error)"=w351, "key"="tdms file", "refnum"=w350) -> ("error out"=w344:errorcluster, "value"=w333:path, "refnum out"=w343:T8)  [unwired: 4 in, 1 out]
        n224 = property on="tdms path" class="Path"(error in=w334, "Value"=w333) -> (error out=w332:errorcluster)  [unwired: 1 in, 1 out]
        n225 = call-poly <vilib>:"Read Key.vi"("section"=w339, "error in (no error)"=w344, "key"="version sheet", "refnum"=w343) -> ("error out"=w341:errorcluster, "value"=w331:path, "refnum out"=w340:T8)  [unwired: 4 in, 1 out]
        n226 = call <vilib>:"Close Config Data.vi"("error in (no error)"=w341, "refnum"=w340) -> ("error out"=w347:errorcluster)  [unwired: 8 in, 1 out]
        n227 = property on="variation sheet" class="Path"(error in=w332, "Value"=w331) -> (error out=w330:errorcluster)  [unwired: 1 in, 1 out]
        n228 = Merge Errors(w347, w330) -> (w337:errorcluster)
        n229 = Merge Errors(w357, w337) -> (w356:errorcluster)
      }
      frame "Idle", Default {
        w378 = T2 {"data"=variant, "state"=enum."Initialize 1"}  # Cluster
        w377 = state."Idle"  # state
        n230 = Bundle By Name(cluster=w378, "state"=w377) -> (w374:T2)
        n231 = Enqueue Element(queue=w376, element=w374, error in (no error)=w373) -> (queue out=w375:refnum<queue>, error out=w371:errorcluster)  [unwired: 1 in, 1 out]
        n232 = Merge Errors(w371) -> (w372:errorcluster)
      }
      frame "Initialize 1" {
        w393 = T2 {"data"=variant, "state"=enum."Initialize 1"}  # Cluster
        w392 = state."Initialize 2"  # state
        n233 = Unbundle By Name(w399) -> ("Names"=w398:refnum<vi>[], "Current Versions"=w397:refnum<vi>[], "New Versions"=w396:refnum<vi>[])
        n234 = for {
          shift-right: [w411] -> w388
          shift-left: w385 -> [w408]
          tunnel: w398 -> [w406] mode=indexing
          tunnel: w397 -> [w405] mode=indexing
          tunnel: w396 -> [w404] mode=indexing
          w407 = FALSE ("Visible")
          n235 = property class="Str"(reference=w406, error in=w408, "Visible"=w407) -> (error out=w410:errorcluster)  [unwired: 1 out]
          n236 = property class="Str"(reference=w405, error in=w408, "Visible"=w407) -> (error out=w409:errorcluster)  [unwired: 1 out]
          n237 = property class="Str"(reference=w404, error in=w408, "Visible"=w407) -> (reference out=w402:refnum<vi>, error out=w401:errorcluster)
          n238 = property class="Str"(reference=w402, error in=w401, "Text.TextColor"=u32 16777222) -> (error out=w400:errorcluster)  [unwired: 1 out]
          n239 = Merge Errors(w410, w409, w400) -> (w411:errorcluster)
        }
        n240 = control-ref of="Run"() -> (w384:refnum<vi>)
        n241 = property class="Bool"(reference=w384, error in=w385, "DisabledEnum"=T7."Disabled and Grayed Out" ("Disabled")) -> (error out=w383:errorcluster)  [unwired: 1 out]
        n242 = Merge Errors(w388, w383) -> (w387:errorcluster)
        n243 = Bundle By Name(cluster=w393, "state"=w392) -> (w391:T2)
        n244 = Enqueue Element(queue=w382, element=w391, error in (no error)=w385) -> (queue out=w381:refnum<queue>, error out=w390:errorcluster)  [unwired: 1 in, 1 out]
        n245 = Merge Errors(w390, w387) -> (w394:errorcluster)
      }
      frame "Initialize 2" {
        w426 = T2 {"data"=variant, "state"=enum."Initialize 1"}  # Cluster
        w425 = state."Read config file"  # state
        n246 = Unbundle By Name(w416) -> ("New Versions"=w418:refnum<vi>[], "keys"=w412:refnum<vi>[])
        n247 = for {
          N: w417 -> [_]
          tunnel: w418 -> [w432] mode=indexing
          shift-right: [w430] -> w413
          shift-left: w415 -> [w431]
          n248 = property class="Str"(reference=w432, error in=w431, "Text.TextColor"=u32 16777222) -> (error out=w430:errorcluster)  [unwired: 1 out]
        }
        n249 = for {
          tunnel: w412 -> [w436] mode=indexing
          shift-right: [w433] -> w419
          shift-left: w415 -> [w434]
          n250 = property class="Bool"(reference=w436, error in=w434, "DisabledEnum"=T7."Enabled" ("Disabled")) -> (error out=w433:errorcluster)  [unwired: 1 out]
        }
        n251 = Bundle By Name(cluster=w426, "state"=w425) -> (w424:T2)
        n252 = property on="Status bar" class="Str"(error in=w419, "Value"="M200: The page was initialized by the latest configuration." ("Status bar")) -> (error out=w414:errorcluster)  [unwired: 1 in, 1 out]
        n253 = Enqueue Element(queue=w421, element=w424, error in (no error)=w415) -> (queue out=w420:refnum<queue>, error out=w423:errorcluster)  [unwired: 1 in, 1 out]
        n254 = Merge Errors(w423, w413, w414) -> (w427:errorcluster)
      }
      frame "Read config file" {
        w444 = T2 {"data"=variant, "state"=enum."Initialize 1"}  # Cluster
        w443 = state."Read TDMS"  # state
        n255 = Bundle By Name(cluster=w444, "state"=w443) -> (w442:T2)
        n256 = Enqueue Element(queue=w439, element=w442, error in (no error)=w441) -> (queue out=w438:refnum<queue>, error out=w440:errorcluster)  [unwired: 1 in, 1 out]
        n257 = call <vilib>:"Is Path and Not Empty.vi"("path"="Config Path") -> ("Is Path and Not Empty?"=w448:bool)  [unwired: 4 in]
        n258 = case shown="True" w448 {
          tunnel: w438 -> [w455 w462]
          tunnel: "Config Path" -> [_ w468]
          tunnel: [w451 w460] -> w447
          tunnel: [0 w456] -> w437
          frame False {
            w454 = T2 {"data"=variant, "state"=enum."Initialize 1"}  # Cluster
            w453 = state."Config file Error"  # state
            n259 = Bundle By Name(cluster=w454, "state"=w453) -> (w452:T2)
            n260 = Enqueue Element At Opposite End(queue=w455, element=w452) -> (error out=w451:errorcluster)  [unwired: 2 in, 2 out]
          }
          frame True {
            w459 = state."Update Comp Names"  # state
            w464 = T2 {"data"=variant, "state"=enum."Initialize 1"}  # Cluster
            n261 = call-poly <vilib>:"Read From Spreadsheet File.vi"("transpose (no:F)"=FALSE, "file path (dialog if empty)"=w468) -> ("all rows"=w466:string[][])  [unwired: 5 in, 4 out]
            n262 = Array Size(array=w466) -> (size(s)=w457:i32[])
            n263 = Bundle("all rows"=w466, w457) -> (w465:cluster{"all rows":string[][], i32[]})  [unwired: 1 in]
            n264 = To Variant(anything=w465) -> (Variant=w463:variant)
            n265 = Index Array(array=w457, index=0) -> (element=w456:i32)
            n266 = Bundle By Name(cluster=w464, "data"=w463, "state"=w459) -> (w461:T2)
            n267 = Enqueue Element(queue=w462, element=w461) -> (error out=w460:errorcluster)  [unwired: 2 in, 2 out]
          }
        }
        n268 = Merge Errors(w440, w447) -> (w449:errorcluster)
      }
      frame "Read TDMS" {
        n269 = call <vilib>:"Is Path and Not Empty.vi"("path"="tdms path") -> ("Is Path and Not Empty?"=w476:bool)  [unwired: 4 in]
        n270 = case shown="False" w476 {
          tunnel: "tdms path" -> [_ w505]
          tunnel: w475 -> [w480 w487]
          tunnel: [w479 w493] -> w470
          tunnel: [w478 w484] -> w473
          tunnel: w472 -> [w478 _]
          frame False {
            w483 = T2 {"data"=variant, "state"=enum."Initialize 1"}  # Cluster
            w482 = state."Config file Error"  # state
            n271 = Bundle By Name(cluster=w483, "state"=w482) -> (w481:T2)
            n272 = Enqueue Element At Opposite End(queue=w480, element=w481) -> (error out=w479:errorcluster)  [unwired: 2 in, 2 out]
          }
          frame True {
            w486 = T2 {"data"=variant, "state"=enum."Initialize 1"}  # Cluster
            w499 = "Version History" ("group name in (Untitled)")
            n273 = TDMS Open(11:w505) -> (0:w504:errorcluster, 3:w503:refnum<k34>)  [unwired: 6 in]
            n274 = TDMS List Contents(4:w504, 6:w499, 7:w503) -> (1:w496:string[], 3:w498:refnum<k34>)  [unwired: 2 out]
            n275 = Array Size(array=w496) -> (size(s)=w495:i32)
            n276 = Reverse 1D Array(array=w496) -> (reversed array=w502:string[])
            n277 = Index Array(array=w502, index=0) -> (element=w500:string)
            n278 = TDMS Read(0:w498, 5:w499, 7:w500, 12:string[] []) -> (4:w484:refnum<k34>, 10:w494:string[])  [unwired: 4 in, 4 out]
            n279 = case shown="1" w495 {
              tunnel: w494 -> [w506 w508]
              tunnel: [w506 w507] -> w491
              frame 2, Default {
              }
              frame 1 {
                n280 = for {
                  tunnel: w508 -> [_] mode=indexing
                  tunnel: ["no records!"] -> w507 mode=indexing
                }
              }
            }
            n281 = Array Size(array=w491) -> (size(s)=w492:i32)
            n282 = Bundle(w491, w492) -> (w490:cluster{string[], i32})  [unwired: 1 in]
            n283 = To Variant(anything=w490) -> (Variant=w489:variant)
            n284 = Bundle By Name(cluster=w486, "state"=state."Update Current Versions", "data"=w489) -> (w485:T2)
            n285 = Enqueue Element(queue=w487, element=w485) -> (error out=w493:errorcluster)  [unwired: 2 in, 2 out]
          }
        }
        n286 = Merge Errors(w474, w470) -> (w477:errorcluster)
      }
      frame "Update Comp Names" {
        w516 = T2 {"data"=variant, "state"=enum."Initialize 1"}  # Cluster
        w515 = state."Idle"  # state
        n287 = Variant To Data(type=cluster{"all rows":string[][], i32[]} {"all rows"=[], []} ("output cluster"), Variant=w526) -> (data=w524:cluster{"all rows":string[][], i32[]})  [unwired: 1 in, 1 out]
        n288 = Unbundle By Name(w513) -> ("Names"=w512:refnum<vi>[])
        n289 = Unbundle(w524) -> ("all rows"=w522:string[][])  [unwired: 1 out]
        n290 = Index Array(array=w522, index (col)=0 ("disabled index (col)")) -> (element=w520:string[])  [unwired: 1 in]
        n291 = for {
          shift-right: [w529] -> w519
          shift-left: w523 -> [w532]
          tunnel: w520 -> [w530] mode=indexing
          tunnel: w512 -> [w527] mode=indexing
          n292 = property class="Str"(reference=w527, error in=w532, "Visible"=TRUE) -> (reference out=w528:refnum<vi>, error out=w531:errorcluster)
          n293 = property class="Str"(reference=w528, error in=w531, "Value"=w530) -> (error out=w529:errorcluster)  [unwired: 1 out]
        }
        n294 = Bundle By Name(cluster=w516, "state"=w515) -> (w514:T2)
        n295 = Enqueue Element(queue=w518, element=w514, error in (no error)=w519) -> (error out=w517:errorcluster)  [unwired: 1 in, 2 out]
      }
      frame "Update Current Versions" {
        w534 = state."Check current versions"  # state
        w545 = T2 {"data"=variant, "state"=enum."Initialize 1"}  # Cluster
        n296 = Unbundle By Name(w540) -> ("Current Versions"=w539:refnum<vi>[], "New Versions"=w538:refnum<vi>[], "Names"=w536:refnum<vi>[])
        n297 = Variant To Data(type=cluster{string[], i32} {[], 0} ("output cluster"), Variant=w549) -> (data=w550:cluster{string[], i32})  [unwired: 1 in, 1 out]
        n298 = Unbundle(w550) -> (w547:string[])  [unwired: 1 out]
        n299 = while {
          shift-right: [w565] -> w543
          shift-left: w546 -> [w558]
          tunnel: w547 -> [w569] mode=indexing
          tunnel: w539 -> [w567] mode=indexing
          tunnel: w538 -> [w564] mode=indexing
          tunnel: w536 -> [w555]
          i -> [w552]
          stop <- w556 continue-if-true
          w563 = TRUE ("Visible")
          n300 = Add(x=1.0, y=w552) -> (x+y=w554:dbl)
          n301 = property class="Str"(reference=w567, error in=w558, "Visible"=w563) -> (reference out=w568:refnum<vi>, error out=w570:errorcluster)
          n302 = property class="Str"(reference=w564, error in=w558, "Visible"=w563) -> (reference out=w562:refnum<vi>, error out=w561:errorcluster)
          n303 = Index Array(array=w555, index=w554) -> (element=w551:refnum<vi>)
          n304 = property class="Str"(reference=w568, error in=w570, "Value"=w569) -> (error out=w566:errorcluster)  [unwired: 1 out]
          n305 = property class="Str"(reference=w562, error in=w561, "Value"="") -> (error out=w560:errorcluster)  [unwired: 1 out]
          n306 = property class="Str"(reference=w551, error in=w558) -> (error out=w557:errorcluster, "Visible"=w556:bool)  [unwired: 1 out]
          n307 = Merge Errors(w566, w560, w557) -> (w565:errorcluster)
        }
        n308 = Bundle By Name(cluster=w545, "state"=w534) -> (w544:T2)
        n309 = Enqueue Element(queue=w542, element=w544, error in (no error)=w543) -> (error out=w541:errorcluster)  [unwired: 1 in, 2 out]
      }
      frame "Make new configuration" {
        w580 = T2 {"data"=variant, "state"=enum."Initialize 1"}  # Cluster
        n310 = Unbundle By Name(w588) -> ("New Versions"=w587:refnum<vi>[], "Current Versions"=w586:refnum<vi>[])
        n311 = Initialize Array "Initialize Array"("", w582) -> (w583:string[])
        n312 = for {
          N: w582 -> [_]
          tunnel: w587 -> [w604] mode=indexing
          tunnel: w586 -> [w610] mode=indexing
          shift-right: [w594] -> w579
          shift-left: w585 -> [w603]
          shift-right: [w602] -> w581
          shift-left: w583 -> [w606]
          shift-right: [w596] -> w574
          shift-left: 0 -> [w597]
          i -> [w605]
          n313 = property class="Str"(reference=w610, error in=w603) -> (error out=w600:errorcluster, "Value"=w609:string)  [unwired: 1 out]
          n314 = property class="Str"(reference=w604, error in=w603) -> (reference out=w598:refnum<vi>, error out=w601:errorcluster, "Value"=w607:string)
          n315 = Merge Errors(w601, w600) -> (w592:errorcluster)
          n316 = Empty String/Path?(string/path=w607) -> (empty?=w608:bool)
          n317 = case shown="False" w608 {
            tunnel: w609 -> [_ w620]
            tunnel: [w617 w620] -> w599
            tunnel: w607 -> [w617 _]
            tunnel: w598 -> [w616 _]
            tunnel: w597 -> [w614 w619]
            tunnel: [w613 w619] -> w596
            tunnel: [w612 w618] -> w593
            tunnel: w592 -> [w611 w618]
            frame False {
              # "new version"
              n318 = Increment(x=w614) -> (x+1=w613:i32)
              n319 = property class="Str"(reference=w616, error in=w611, "Text.TextColor"=u32 16714752) -> (error out=w612:errorcluster)  [unwired: 1 out]
            }
            frame True {
              # "no new version"
            }
          }
          n320 = property class="Str"(reference=w598, error in=w592, "Value"=w599) -> (error out=w595:errorcluster)  [unwired: 1 out]
          n321 = Replace Array Subset(array=w606, new element=w599, index=w605) -> (w602:string[])
          n322 = Merge Errors(w595, w593) -> (w594:errorcluster)
        }
        n323 = Equal To 0?(x=w574) -> (x = 0?=w573:bool)
        n324 = case shown="True" w573 {
          tunnel: [w590 w591] -> w571
          frame False {
            w590 = state."Register Change"  # state
            # "There is at least one new version"
          }
          frame True {
            w591 = state."No New Update"  # state
            # "No New Updates"
          }
        }
        n325 = To Variant(anything=w581) -> (Variant=w572:variant)
        n326 = Bundle By Name(cluster=w580, "state"=w571, "data"=w572) -> (w577:T2)
        n327 = Enqueue Element(queue=w576, element=w577, error in (no error)=w579) -> (error out=w578:errorcluster)  [unwired: 1 in, 2 out]
      }
      frame "Register Change" {
        n328 = Variant To Data(error in=w632, type=string[] [], Variant=w633) -> (data=w630:string[], error out=w625:errorcluster)
        n329 = call "Confirm changes"("error in (no error)"=w625) -> ("Sign with your name"=w622:string, "Confirm"=w623:bool, "error out"=w624:errorcluster)  [unwired: 16 in]
        n330 = case shown="False" w623 {
          tunnel: w629 -> [_ w645]
          tunnel: w624 -> [w634 w647]
          tunnel: w630 -> [_ w655]
          tunnel: [w635 w650] -> w628
          tunnel: w627 -> [w640 w651]
          tunnel: ["M400: The configuration was rejected." ("F button name (\"Cancel\")") "M300: The configuration was successfully registered. Refresh the page to continue." ("F button name (\"Cancel\")")] -> w626
          tunnel: w622 -> [_ w642]
          frame False {
            w639 = T2 {"data"=variant, "state"=enum."Initialize 1"}  # Cluster
            w638 = state."Idle"  # state
            n331 = Bundle By Name(cluster=w639, "state"=w638) -> (w637:T2)
            n332 = Enqueue Element(queue=w640, element=w637, error in (no error)=w634) -> (error out=w635:errorcluster)  [unwired: 1 in, 2 out]
          }
          frame True {
            w654 = T2 {"data"=variant, "state"=enum."Initialize 1"}  # Cluster
            w653 = state."Idle"  # state
            n333 = Build Array(w642) -> (w641:string[])
            n334 = Get Date/Time In Seconds() -> (seconds since 1Jan1904=w656:timestamp)
            n335 = Format Date/Time String(time format string (%c)="Date: %Y-%b-%d    Time: %H:%M:%S", seconds (now)=w656) -> (date/time string=w643:string)  [unwired: 1 in]
            n336 = TDMS Write(0:w645, 5:"Reporter" ("group name in (Untitled)"), 7:w643, 9:w641, 11:w647) -> (15:w646:errorcluster)  [unwired: 1 in, 3 out]
            n337 = TDMS Write(0:w645, 5:"Version History" ("group name in (Untitled)"), 7:w643, 9:w655, 11:w646) -> (15:w649:errorcluster)  [unwired: 1 in, 3 out]
            n338 = Bundle By Name(cluster=w654, "state"=w653) -> (w652:T2)
            n339 = Enqueue Element(queue=w651, element=w652, error in (no error)=w649) -> (error out=w650:errorcluster)  [unwired: 1 in, 2 out]
          }
        }
        "Status bar" <- w626
      }
      frame "View Registry" {
        w664 = T2 {"data"=variant, "state"=enum."Initialize 1"}  # Cluster
        w663 = state."Idle"  # state
        n340 = property on="tdms path" class="Path"(error in=w667) -> (error out=w665:errorcluster, "Value"=w666:path)  [unwired: 1 in, 1 out]
        n341 = call <vilib>:"TDMS - File Viewer.vi"("error in (no error)"=w665, "file path"=w666) -> ("error out"=w660:errorcluster)  [unwired: 4 in, 1 out]
        n342 = Bundle By Name(cluster=w664, "state"=w663) -> (w661:T2)
        n343 = Enqueue Element(queue=w662, element=w661, error in (no error)=w660) -> (error out=w659:errorcluster)  [unwired: 1 in, 2 out]
      }
      frame "Add Comment" {
        n344 = call "Comment"("error in (no error)"=w682) -> ("Name"=w678:string, "Comment"=w677:string, "Add"=w684:bool, "error out"=w673:errorcluster)  [unwired: 15 in]
        n345 = TDMS List Contents(4:w682, 6:"Version History" ("group name in (Untitled)"), 7:w676) -> (0:w672:errorcluster, 1:w670:string[], 3:w686:refnum<k34>)  [unwired: 1 out]
        n346 = Merge Errors(w673, w672) -> (w683:errorcluster)
        n347 = Build Array(w678, w677) -> (w674:string[])
        n348 = case shown="True" w684 {
          tunnel: w686 -> [w690 w700]
          tunnel: w683 -> [w689 w699]
          tunnel: [w690 w698] -> w685
          tunnel: [w689 w697] -> w681
          tunnel: w674 -> [_ w693]
          tunnel: "Comment" ("group name in (Untitled)") -> [_ w691]
          tunnel: w670 -> [_ w694]
          frame False {
          }
          frame True {
            n349 = Reverse 1D Array(array=w694) -> (reversed array=w695:string[])
            n350 = Index Array(array=w695, index=0) -> (element=w692:string)
            n351 = TDMS Write(0:w700, 5:w691, 7:w692, 9:w693, 11:w699) -> (4:w698:refnum<k34>, 15:w697:errorcluster)  [unwired: 1 in, 2 out]
          }
        }
        n352 = property on="Status bar" class="Str"(error in=w681, "Value"="M500: Comment was successfully added to the latest entry." ("Status bar")) -> (error out=w679:errorcluster)  [unwired: 1 in, 1 out]
      }
      frame "No New Update" {
        w706 = T2 {"data"=variant, "state"=enum."Initialize 1"}  # Cluster
        w701 = state."Initialize 2"  # state
        n353 = flat-sequence {
          tunnel: w707 -> [w713]
          tunnel: [w713] -> w705
          tunnel: [w710] -> _
          frame #0 {
            n354 = One Button Dialog(message="There is no new updates. To register a new configuration, you need at least one new version.\nThe page will be reinitialized with the latest configuration.", button name ("OK")="OK") -> (true=w710:bool)
          }
        }
        n355 = Bundle By Name(cluster=w706, "state"=w701) -> (w702:T2)
        n356 = Enqueue Element(queue=w704, element=w702, error in (no error)=w705) -> (error out=w703:errorcluster)  [unwired: 1 in, 2 out]
      }
      frame "Check current versions" {
        n357 = Unbundle By Name(w717) -> ("Current Versions"=w716:refnum<vi>[])
        n358 = for {
          N: w718 -> [_]
          tunnel: w716 -> [w727] mode=indexing
          shift-right: [w722] -> w714
          shift-left: w715 -> [w726]
          n359 = property class="Str"(reference=w727, error in=w726) -> (reference out=w721:refnum<vi>, error out=w723:errorcluster, "Value"=w725:string)
          n360 = Empty String/Path?(string/path=w725) -> (empty?=w724:bool)
          n361 = case shown="True" w724 {
            tunnel: w723 -> [w728 _]
            tunnel: [w728 w731] -> w722
            tunnel: w721 -> [_ w730]
            frame False {
              # "version exits"
            }
            frame True {
              n362 = property class="Str"(reference=w730, "Value"="no records!") -> (error out=w731:errorcluster)  [unwired: 1 in, 1 out]
            }
          }
        }
      }
      frame "Config file Error" {
        n363 = One Button Dialog(message="Error in (txt or tdms) file path.\nEither Not A Path or Path is Empty.", button name ("OK")="Close Application") -> (true=w737:bool)
        n364 = case shown="True" w737 {
          tunnel: w732 -> [_ w740]
          frame False {
          }
          frame True {
            w741 = T2 {"data"=variant, "state"=enum."Initialize 1"}  # Cluster
            w742 = state."Close"  # state
            n365 = Bundle By Name(cluster=w741, "state"=w742) -> (w739:T2)
            n366 = Enqueue Element At Opposite End(queue=w740, element=w739) -> ()  [unwired: 2 in, 3 out]
          }
        }
      }
      frame "Write ini file" {
        w761 = T2 {"data"=variant, "state"=enum."Initialize 1"}  # Cluster
        w762 = state."Close"  # state
        w744 = "Path" ("section")
        n367 = Current VI's Path() -> (path=w754:path)
        n368 = disable-structure shown="RUN_TIME_ENGINE==True" {
          disable-tunnel: w754 -> [w779 w783]
          disable-tunnel: [w778 w780] -> w753
          frame condition #0 (active) {
            n369 = Strip Path(path=w779) -> (stripped path=w778:path)  [unwired: 1 out]
          }
          frame condition #1 {
            n370 = Strip Path(path=w783) -> (stripped path=w782:path)  [unwired: 1 out]
            n371 = Strip Path(path=w782) -> (stripped path=w781:path)  [unwired: 1 out]
            n372 = Strip Path(path=w781) -> (stripped path=w780:path)  [unwired: 1 out]
          }
        }
        n373 = Build Path(base path=w753, name or relative path=w743) -> (appended path=w775:path)
        n374 = property on="Config Path" class="Path"(error in=w758) -> (error out=w766:errorcluster, "Value"=w765:path)  [unwired: 1 in, 1 out]
        n375 = call <vilib>:"Open Config Data.vi"("error in (no error)"=w758, "create file if necessary (T)"=FALSE, "configuration file path"=w775) -> ("error out"=w773:errorcluster, "refnum"=w774:T8)  [unwired: 6 in, 1 out]
        n376 = call-poly <vilib>:"Write Key.vi"("section"=w744, "error in (no error)"=w773, "value"=w765, "key"="txt config file", "refnum"=w774) -> ("error out"=w771:errorcluster, "refnum out"=w770:T8)  [unwired: 4 in, 1 out]
        n377 = property on="tdms path" class="Path"(error in=w766) -> (error out=w750:errorcluster, "Value"=w764:path)  [unwired: 1 in, 1 out]
        n378 = call-poly <vilib>:"Write Key.vi"("section"=w744, "error in (no error)"=w771, "value"=w764, "key"="tdms file", "refnum"=w770) -> ("error out"=w752:errorcluster, "refnum out"=w751:T8)  [unwired: 4 in, 1 out]
        n379 = property on="variation sheet" class="Path"(error in=w750) -> (error out=w747:errorcluster, "Value"=w749:path)  [unwired: 1 in, 1 out]
        n380 = call-poly <vilib>:"Write Key.vi"("section"=w744, "error in (no error)"=w752, "value"=w749, "key"="version sheet", "refnum"=w751) -> ("error out"=w746:errorcluster, "refnum out"=w745:T8)  [unwired: 4 in, 1 out]
        n381 = call <vilib>:"Close Config Data.vi"("error in (no error)"=w746, "refnum"=w745) -> ("error out"=w767:errorcluster)  [unwired: 8 in, 1 out]
        n382 = Merge Errors(w767, w747) -> (w755:errorcluster)
        n383 = Bundle By Name(cluster=w761, "state"=w762) -> (w756:T2)
        n384 = Enqueue Element(queue=w760, element=w756, error in (no error)=w758) -> (queue out=w759:refnum<queue>, error out=w757:errorcluster)  [unwired: 1 in, 1 out]
        n385 = Merge Errors(w757, w755) -> (w763:errorcluster)
      }
      frame "Close" {
        n386 = Unbundle By Name(w789) -> ("Names"=w788:refnum<vi>[], "Current Versions"=w787:refnum<vi>[], "New Versions"=w786:refnum<vi>[])
        n387 = control-ref of="Run"() -> (w796:refnum<vi>)
        n388 = property class="Bool"(reference=w796, error in=w794, "DisabledEnum"=T7."Enabled" ("Disabled")) -> (error out=w793:errorcluster)  [unwired: 1 out]
        n389 = for {
          N: w784 -> [_]
          shift-right: [w812] -> w785
          shift-left: _ -> [w809]
          tunnel: w788 -> [w806] mode=indexing
          tunnel: w787 -> [w805] mode=indexing
          tunnel: w786 -> [w804] mode=indexing
          w808 = FALSE ("Visible")
          n390 = property class="Str"(reference=w806, error in=w809, "Visible"=w808) -> (error out=w811:errorcluster)  [unwired: 1 out]
          n391 = property class="Str"(reference=w805, error in=w809, "Visible"=w808) -> (error out=w810:errorcluster)  [unwired: 1 out]
          n392 = property class="Str"(reference=w804, error in=w809, "Visible"=w808) -> (error out=w807:errorcluster)  [unwired: 1 out]
          n393 = Merge Errors(w811, w810, w807) -> (w812:errorcluster)
        }
        n394 = Release Queue(queue=w803, error in (no error)=w794) -> (error out=w802:errorcluster)  [unwired: 1 in, 2 out]
        n395 = TDMS Close(8:w794, 11:w797) -> (0:w798:errorcluster)  [unwired: 1 out]
        n396 = property on="Status bar" class="Str"(error in=w793, "Value"="M700: Application ended." ("Status bar")) -> (error out=w792:errorcluster)  [unwired: 1 in, 1 out]
        n397 = Merge Errors(w802, w798, w792, w785) -> (w801:errorcluster)
        n398 = disable-structure shown="Default" {
          disable-tunnel: w801 -> [w814 w816]
          disable-tunnel: [w814 w816] -> w800
          disable-tunnel: TRUE ("quit? (T)") -> [w813 w815]
          frame condition #0 (active) {
            n399 = Stop(stop? (T)=w813) -> ()
          }
          frame condition #1 {
            n400 = Quit LabVIEW(quit? (T)=w815) -> ()
          }
        }
      }
      frame "Read Variation Sheet" {
        w824 = T2 {"data"=variant, "state"=enum."Initialize 1"}  # Cluster
        w825 = state."Search and write current versions"  # state
        n401 = call <vilib>:"Open Config Data.vi"("error in (no error)"=w820, "create file if necessary (T)"=FALSE, "configuration file path"="variation sheet") -> ("error out"=w831:errorcluster, "refnum"=w830:T8)  [unwired: 6 in, 1 out]
        n402 = call <vilib>:"Get Section Names.vi"("error in (no error)"=w831, "refnum"=w830) -> ("error out"=w829:errorcluster, "section names"=w827:string[], "refnum out"=w828:T8)  [unwired: 7 in]
        n403 = for {
          tunnel: w827 -> [w838] mode=indexing
          shift-right: [w837] -> w818
          shift-left: w829 -> [w842]
          tunnel: w828 -> [w843]
          tunnel: [w836] -> w817
          n404 = call <vilib>:"Get Key Names.vi"("section"=w838, "error in (no error)"=w842, "refnum"=w843) -> ("error out"=w839:errorcluster, "key names"=w840:string[], "refnum out"=w841:T8)  [unwired: 5 in, 1 out]
          n405 = for {
            tunnel: w841 -> [w851]
            tunnel: w840 -> [w845] mode=indexing
            shift-right: [w849] -> w837
            shift-left: w839 -> [w850]
            tunnel: w838 -> [w847]
            tunnel: [w848] -> _ mode=indexing
            tunnel: [w846] -> w836 mode=indexing
            n406 = call-poly <vilib>:"Read Key.vi"("section"=w847, "error in (no error)"=w850, "key"=w845, "refnum"=w851) -> ("error out"=w849:errorcluster, "value"=w844:string, "refnum out"=w848:T8)  [unwired: 4 in, 1 out]
            n407 = Build Array(w847, w845, w844) -> (w846:string[])
          }
        }
        n408 = To Variant(anything=w817) -> (Variant=w823:variant)
        n409 = Bundle By Name(cluster=w824, "data"=w823, "state"=w825) -> (w826:T2)
        n410 = Enqueue Element(queue=w822, element=w826, error in (no error)=w818) -> (queue out=w821:refnum<queue>, error out=w819:errorcluster)  [unwired: 1 in, 1 out]
      }
      frame "Search and write current versions" {
        n411 = Unbundle By Name(w858) -> ("Names"=w857:refnum<vi>[], "New Versions"=w856:refnum<vi>[], "Current Versions"=w855:refnum<vi>[])
        n412 = Variant To Data(error in=w853, type=string[][] [], Variant=w862) -> (data=w859:string[][])  [unwired: 1 out]
        n413 = Index Array(array=w859, index (col)=0 ("index (row)")) -> ()  [unwired: 1 in, 1 out]
        n414 = for {
          N: w854 -> [_]
          tunnel: w859 -> [w876]
          tunnel: w857 -> [w868]
          tunnel: w856 -> [w877]
          tunnel: w855 -> [w875]
          shift-right: [w865] -> w852
          shift-left: w853 -> [w870]
          i -> [w867]
          n415 = Index Array(array=w868, index=w867) -> (element=w866:refnum<vi>)
          n416 = property class="Str"(reference=w866, error in=w870) -> (error out=w869:errorcluster, "Value"=w874:string)  [unwired: 1 out]
          n417 = Index Array(array=w876, index (col)=1 ("disabled index (col)")) -> (element=w873:string[])  [unwired: 1 in]
          n418 = for {
            tunnel: w873 -> [w882] mode=indexing
            tunnel: w874 -> [w881]
            tunnel: [w880] -> w872
            tunnel: [w879] -> w871
            i -> [w880]
            stop <- w879 stop-if-true
            n419 = Equal?(x=w882, y=w881) -> (x = y?=w879:bool)
          }
          n420 = Array Size(array=w873) -> ()  [unwired: 1 out]
          n421 = case shown="True" w871 {
            tunnel: w877 -> [_ w897]
            tunnel: w876 -> [_ w895]
            tunnel: w875 -> [_ w893]
            tunnel: w872 -> [_ w888]
            tunnel: w867 -> [_ w887]
            tunnel: w869 -> [w883 w886]
            tunnel: [w883 w884] -> w865
            frame False {
            }
            frame True {
              n422 = Index Array(array=w897, index=w887) -> (element=w896:refnum<vi>)
              n423 = Index Array(array=w893, index=w887) -> (element=w892:refnum<vi>)
              n424 = property class="Str"(reference=w892, error in=w886) -> (error out=w885:errorcluster, "Value"=w891:string)  [unwired: 1 out]
              n425 = Index Array(array=w895, index (row)=w888, index (col)=2 ("disabled index (col)")) -> (element=w890:string)
              n426 = Not Equal?(x=w890, y=w891) -> (x != y?=w889:bool)
              n427 = case shown="True" w889 {
                tunnel: w896 -> [_ w905]
                tunnel: w890 -> [_ w902]
                tunnel: w885 -> [w898 w901]
                tunnel: [w898 w899] -> w884
                frame False {
                }
                frame True {
                  n428 = property class="Str"(reference=w905, error in=w901, "Value"=w902) -> (reference out=w904:refnum<vi>, error out=w900:errorcluster)
                  n429 = property class="Str"(reference=w904, error in=w900, "Text.TextColor"=u32 1985280) -> (error out=w899:errorcluster)  [unwired: 1 out]
                }
              }
            }
          }
        }
      }
    }
  }
  n430 = Release Queue(queue=w40, error in (no error)=w41) -> (error out=w39:errorcluster)  [unwired: 1 in, 2 out]
  n431 = call <vilib>:"Simple Error Handler.vi"("error in (no error)"=w39) -> ()  [unwired: 4 in, 5 out]
